vi "niRFUtil FTW Compute RBW and Sweep Time.vi"(0 "RBW Filter":T7={"Auto Bandwidth"=enum."True", "Type"=enum."Gaussian", "Bandwidth (Hz)"=100000.0, "Bandwidth Definition"=enum."3dB"} {"Bandwidth (Hz)" format="%^.3e"}, 5 "Sweep Time":T4={"Auto"=enum."True", "Interval (s)"=0.001} {"Interval (s)" format="%^.2e"}, 7 "FFT":T10={"Window"=enum."Flat Top", "Padding"=1.0} {"Padding" min=1.0 format="%.2f"}, 9 "IBW or Span (Hz)":dbl=1000000.0 format="%.3e", 12 "(IBW or Span)/RBW":dbl=100.0, 13 "RBW/Bin Size":dbl=10.0, 14 "Max DIBW (Hz)":dbl=inf format="%.3e") -> (3 "System RBW":T1={"Type"=enum."Gaussian", "Bandwidth (Hz)"=100000.0} {"Bandwidth (Hz)" format="%^.3e"}, 4 "RBW Filter Out":T7={"Auto Bandwidth"=enum."True", "Type"=enum."Gaussian", "Bandwidth (Hz)"=100000.0, "Bandwidth Definition"=enum."3dB"} {"Bandwidth (Hz)" format="%^.3e"}, 6 "Sweep Time Out":T4={"Auto"=enum."True", "Interval (s)"=0.001} {"Interval (s)" format="%^.2e"})   [LabVIEW 2015, in "niRFUtil.lvlib"]
uses:
  niRFUtil.lvlib
  Includes/niRFUtil INC RBW Filter (Freq Domain).ctl
  Includes/niRFUtil INC RBW Auto.ctl
  Includes/niRFUtil INC RBW Filter Type (Freq Domain).ctl
  Includes/niRFUtil INC RBW Filter Bandwidth.ctl
  Includes/niRFUtil INC Bandwidth Definition.ctl
  Includes/niRFUtil INC Sweep Time.ctl
  Includes/niRFUtil INC Sweep Time Auto.ctl
  Includes/niRFUtil INC Sweep Time Interval.ctl
  Includes/niRFUtil INC FFT.ctl
  Includes/niRFUtil INC FFT Window.ctl
  Includes/niRFUtil INC FFT Padding.ctl
  Includes/System/niRFUtil INC System RBW Filter (Frequency Domain).ctl
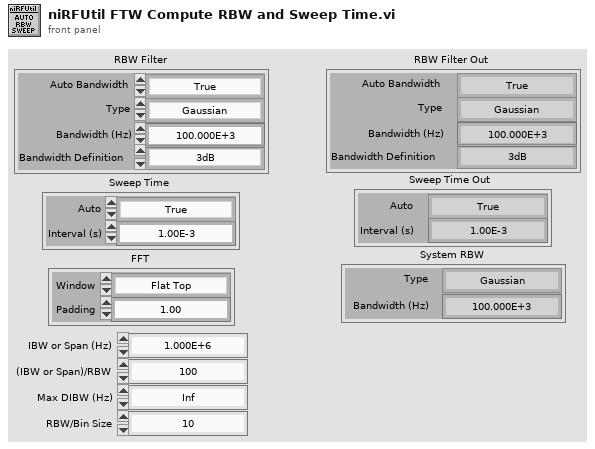
[diagram p1: front panel]
types:
  T1 = typedef "niRFUtil.lvlib/niRFUtil INC System RBW Filter (Frequency Domain).ctl" = cluster{"Type":T2, "Bandwidth (Hz)":T3}
  T2 = typedef "niRFUtil.lvlib/niRFUtil INC RBW Filter Type (Freq Domain).ctl" = enum16{"FFT Based", "Gaussian", "Flat", "Synch Tuned - 4", "Synch Tuned - 5"}
  T3 = typedef "niRFUtil.lvlib/niRFUtil INC RBW Filter Bandwidth.ctl" = dbl
  T4 = typedef "niRFUtil.lvlib/niRFUtil INC Sweep Time.ctl" = cluster{"Auto":T5, "Interval (s)":T6}
  T5 = typedef "niRFUtil.lvlib/niRFUtil INC Sweep Time Auto.ctl" = enum16{"False", "True"}
  T6 = typedef "niRFUtil.lvlib/niRFUtil INC Sweep Time Interval.ctl" = dbl
  T7 = typedef "niRFUtil.lvlib/niRFUtil INC RBW Filter (Freq Domain).ctl" = cluster{"Auto Bandwidth":T8, "Type":T2, "Bandwidth (Hz)":T3, "Bandwidth Definition":T9}
  T8 = typedef "niRFUtil.lvlib/niRFUtil INC RBW Auto.ctl" = enum16{"False", "True"}
  T9 = typedef "niRFUtil.lvlib/niRFUtil INC Bandwidth Definition.ctl" = enum16{"3dB", "6dB", "Bin Width", "ENBW"}
  T10 = typedef "niRFUtil.lvlib/niRFUtil INC FFT.ctl" = cluster{"Window":T11, "Padding":T12}
  T11 = typedef "niRFUtil.lvlib/niRFUtil INC FFT Window.ctl" = enum16{"None", "Flat Top", "Hanning", "Hamming", "Gaussian", "Blackman", "Blackman-Harris", "Kaiser-Bessel 70 dB", "Kaiser-Bessel 90 dB", "Kaiser-Bessel 110 dB"}
  T12 = typedef "niRFUtil.lvlib/niRFUtil INC FFT Padding.ctl" = dbl
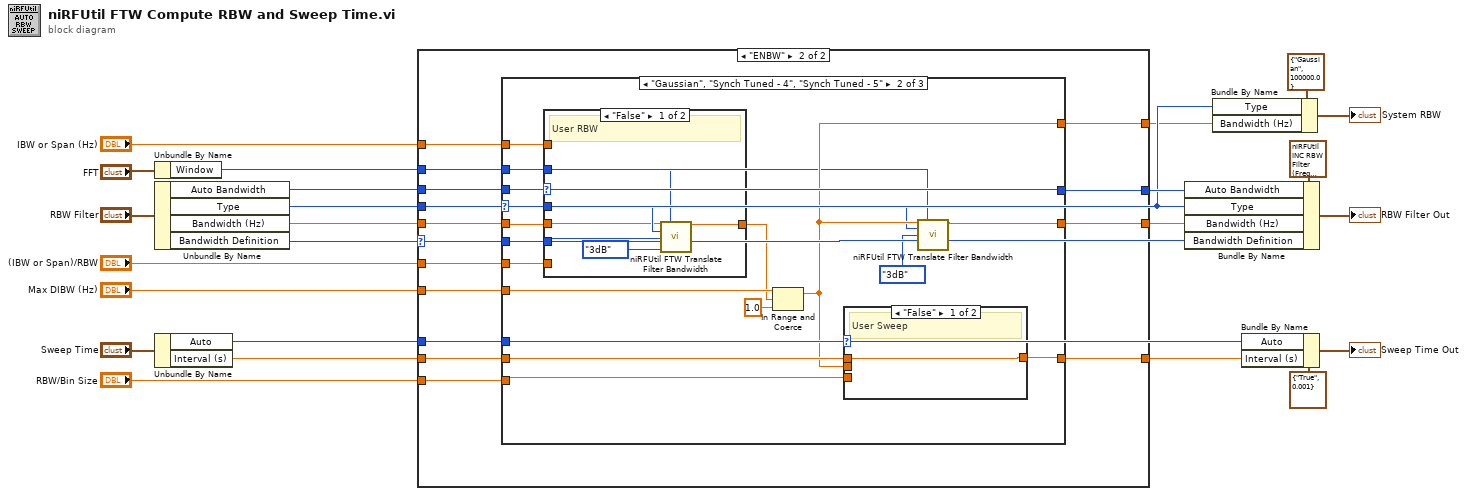
[diagram p0: block diagram]
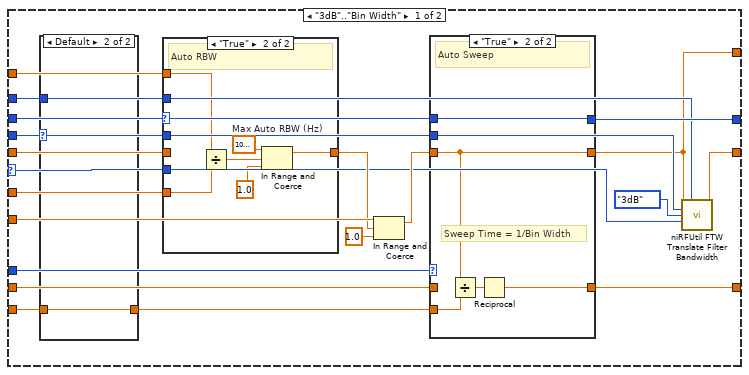
[diagram p2: hidden frame]
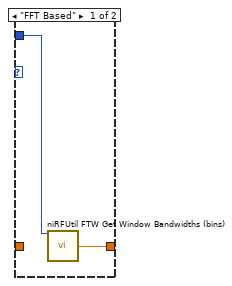
[diagram p3: hidden frame]
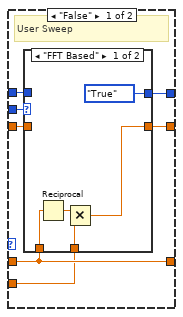
[diagram p4: hidden frame]
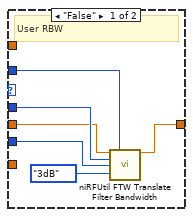
[diagram p6: hidden frame]
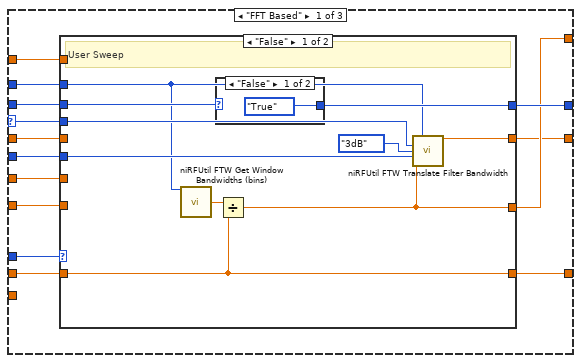
[diagram p7: hidden frame]
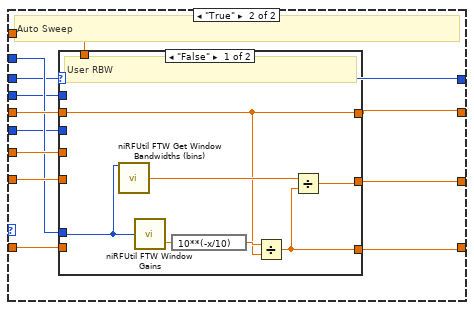
[diagram p9: hidden frame]
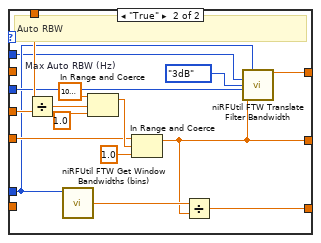
[diagram p10: hidden frame]
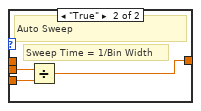
[diagram p11: hidden frame]
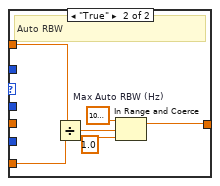
[diagram p12: hidden frame]
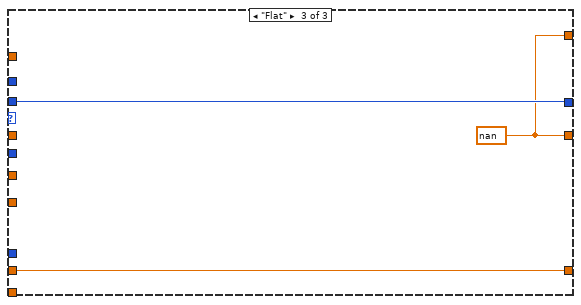
[diagram p13: hidden frame]
diagram:
  n1 = Unbundle By Name("FFT") -> ("Window"=w8:T11)
  n2 = Unbundle By Name("RBW Filter") -> ("Auto Bandwidth"=w10:T8, "Type"=w5:T2, "Bandwidth (Hz)"=w2:T3, "Bandwidth Definition"=w1:T9)
  n3 = Unbundle By Name("Sweep Time") -> ("Auto"=w3:T5, "Interval (s)"=w14:T6)
  n4 = case shown="\"ENBW\"" w1 {
    selector: w1 -> [w25 w79]
    tunnel: "IBW or Span (Hz)" -> [w44 w81]
    tunnel: "RBW/Bin Size" -> [w43 w82]
    tunnel: "(IBW or Span)/RBW" -> [w42 w84]
    tunnel: "Max DIBW (Hz)" -> [w41 w85]
    tunnel: w2 -> [w40 w80]
    tunnel: w14 -> [w39 w90]
    tunnel: w3 -> [w37 w91]
    tunnel: [w36 w89] -> w11
    tunnel: w10 -> [w35 w88]
    tunnel: [w34 w87] -> w9
    tunnel: w8 -> [w33 w92]
    tunnel: [w31 w83] -> w7
    tunnel: w5 -> [w30 w93]
    tunnel: [w29 w86] -> w4
    frame "3dB".."Bin Width" {
      n5 = case shown="Default" w30 {
        tunnel: w43 -> [_ w47]
        tunnel: [w46 w47] -> w38
        tunnel: w33 -> [w45 _]
        frame "FFT Based" {
          n6 = call "niRFUtil FTW Get Window Bandwidths (bins).vi"("FFT Window"=w45) -> ("Bins (3dB)"=w46:dbl)  [unwired: 12 in, 2 out]
        }
        frame Default {
        }
      }
      n7 = case shown="\"True\"" w35 {
        tunnel: [w68 w76] -> w28
        tunnel: w40 -> [w69 _]
        tunnel: w44 -> [_ w78]
        tunnel: w42 -> [_ w77]
        tunnel: w30 -> [w71 _]
        tunnel: w25 -> [w72 _]
        tunnel: w33 -> [w70 _]
        frame "False" {
          # "User RBW"
          n8 = call "niRFUtil FTW Translate Filter Bandwidth.vi"("Input Bandwidth (Hz)"=w69, "FFT Window"=w70, "Filter Type"=w71, "Input Bandwidth Definition"=w72, "Output Bandwidth Definition"=niRFUtil_INC_Bandwidth_Definition."3dB" ("Bandwidth Definition")) -> ("Output Bandwidth (Hz)"=w68:T3)  [unwired: 10 in]
        }
        frame "True" {
          w73 = 1000000.0  # Max Auto RBW (Hz)
          # "Auto RBW"
          n9 = Divide(x=w78, y=w77) -> (x/y=w75:dbl)
          n10 = In Range and Coerce(upper limit=w73, x=w75, lower limit=1.0) -> (coerced(x)=w76:dbl)  [unwired: 1 out]
        }
      }
      n11 = In Range and Coerce(upper limit=w41, x=w28, lower limit=1.0) -> (coerced(x)=w26:T3)  [unwired: 1 out]
      n12 = case shown="\"True\"" w37 {
        tunnel: w39 -> [w49 _]
        tunnel: w38 -> [w48 w66]
        tunnel: w26 -> [w51 w62]
        tunnel: [w49 w64] -> w36
        tunnel: w30 -> [w54 _]
        tunnel: w35 -> [w53 w63]
        tunnel: [w52 w63] -> w34
        tunnel: [w50 w62] -> w29
        frame "False" {
          # "User Sweep"
          n13 = case shown="\"FFT Based\"" w54 {
            tunnel: w53 -> [_ w61]
            tunnel: [niRFUtil_INC_RBW_Auto."True" ("Auto Bandwidth") w61] -> w52
            tunnel: w51 -> [_ w60]
            tunnel: [w55 w60] -> w50
            tunnel: w49 -> [w58 _]
            tunnel: w48 -> [w56 _]
            frame "FFT Based" {
              n14 = Reciprocal(x=w58) -> (1/x=w57:T6)
              n15 = Multiply(x=w57, y=w56) -> (x*y=w55:T6)
            }
            frame Default {
            }
          }
        }
        frame "True" {
          # "Sweep Time = 1/Bin Width"
          # "Auto Sweep"
          n16 = Divide(x=w62, y=w66) -> (x/y=w65:T3)
          n17 = Reciprocal(x=w65) -> (1/x=w64:T3)
        }
      }
      n18 = call "niRFUtil FTW Translate Filter Bandwidth.vi"("Input Bandwidth (Hz)"=w29, "FFT Window"=w33, "Filter Type"=w30, "Input Bandwidth Definition"=niRFUtil_INC_Bandwidth_Definition."3dB", "Output Bandwidth Definition"=w25) -> ("Output Bandwidth (Hz)"=w31:T3)  [unwired: 10 in]
    }
    frame "ENBW" {
      n19 = case shown="\"Gaussian\", \"Synch Tuned - 4\", \"Synch Tuned - 5\"" w93 {
        selector: w93 -> [w96 w155 _]
        tunnel: w92 -> [w102 w156 _]
        tunnel: w91 -> [w107 w167 _]
        tunnel: w90 -> [w106 w166 w188]
        tunnel: [w105 w165 w188] -> w89
        tunnel: w88 -> [w104 w161 w190]
        tunnel: [w103 w161 w190] -> w87
        tunnel: [w101 w158 w189] -> w86
        tunnel: w80 -> [w100 w168 _]
        tunnel: w85 -> [w99 w170 _]
        tunnel: w84 -> [w98 w162 _]
        tunnel: w79 -> [w97 w157 _]
        tunnel: [w95 w159 w189] -> w83
        tunnel: w82 -> [_ w164 _]
        tunnel: w81 -> [w94 w163 _]
        frame "FFT Based" {
          n20 = case shown="\"False\"" w107 {
            tunnel: [w115 w126] -> w105
            tunnel: w106 -> [w115 w125]
            tunnel: w104 -> [w117 w124]
            tunnel: w102 -> [w109 w128]
            tunnel: [w111 w124] -> w103
            tunnel: [w108 w127] -> w101
            tunnel: w100 -> [_ w131]
            tunnel: w99 -> [_ w129]
            tunnel: w98 -> [_ w130]
            tunnel: w97 -> [w113 w121]
            tunnel: w96 -> [w112 w120]
            tunnel: [w110 w122] -> w95
            tunnel: w94 -> [_ w123]
            frame "False" {
              # "User Sweep"
              n21 = call "niRFUtil FTW Get Window Bandwidths (bins).vi"("FFT Window"=w109) -> ("Bins (3dB)"=w116:dbl)  [unwired: 12 in, 2 out]
              n22 = case shown="\"False\"" w117 {
                selector: w117 -> [_ w119]
                tunnel: [niRFUtil_INC_RBW_Auto."True" ("Auto Bandwidth") w119] -> w111
                frame "False" {
                }
                frame "True" {
                  # "Auto RBW"
                }
              }
              n23 = Divide(x=w116, y=w115) -> (x/y=w108:T6)
              n24 = call "niRFUtil FTW Translate Filter Bandwidth.vi"("Input Bandwidth (Hz)"=w108, "FFT Window"=w109, "Filter Type"=w112, "Input Bandwidth Definition"=niRFUtil_INC_Bandwidth_Definition."3dB", "Output Bandwidth Definition"=w113) -> ("Output Bandwidth (Hz)"=w110:T3)  [unwired: 10 in]
            }
            frame "True" {
              # "Auto Sweep"
              n25 = case shown="\"False\"" w124 {
                tunnel: w131 -> [w133 _]
                tunnel: w130 -> [_ w151]
                tunnel: w129 -> [_ w148]
                tunnel: w128 -> [w135 w141]
                tunnel: [w134 w139] -> w127
                tunnel: [w132 w146] -> w126
                tunnel: w125 -> [_ _]
                tunnel: w123 -> [_ w145]
                tunnel: [w133 w143] -> w122
                tunnel: w121 -> [_ w142]
                tunnel: w120 -> [_ w140]
                frame "False" {
                  # "User RBW"
                  n26 = call "niRFUtil FTW Get Window Bandwidths (bins).vi"("FFT Window"=w135) -> ("Bins (3dB)"=w136:dbl)  [unwired: 12 in, 2 out]
                  n27 = call "niRFUtil FTW Window Gains.vi"("Window"=w135) -> ("-ENBW (dB-Hz)"=w138:sgl)  [unwired: 2 in, 1 out]
                  n28 = expression code="10**(-x/10)"(w138) -> (w137:sgl)
                  n29 = Divide(x=w137, y=w133) -> (x/y=w132:T3)
                  n30 = Divide(x=w136, y=w132) -> (x/y=w134:T3)
                }
                frame "True" {
                  w152 = 1000000.0  # Max Auto RBW (Hz)
                  # "Auto RBW"
                  n31 = Divide(x=w145, y=w151) -> (x/y=w154:dbl)
                  n32 = call "niRFUtil FTW Get Window Bandwidths (bins).vi"("FFT Window"=w141) -> ("Bins (3dB)"=w147:dbl)  [unwired: 12 in, 2 out]
                  n33 = In Range and Coerce(upper limit=w152, x=w154, lower limit=1.0) -> (coerced(x)=w149:dbl)  [unwired: 1 out]
                  n34 = In Range and Coerce(upper limit=w148, x=w149, lower limit=1.0) -> (coerced(x)=w139:dbl)  [unwired: 1 out]
                  n35 = Divide(x=w147, y=w139) -> (x/y=w146:dbl)
                  n36 = call "niRFUtil FTW Translate Filter Bandwidth.vi"("Input Bandwidth (Hz)"=w139, "FFT Window"=w141, "Filter Type"=w140, "Input Bandwidth Definition"=niRFUtil_INC_Bandwidth_Definition."3dB", "Output Bandwidth Definition"=w142) -> ("Output Bandwidth (Hz)"=w143:T3)  [unwired: 10 in]
                }
              }
            }
          }
        }
        frame "Gaussian", "Synch Tuned - 4", "Synch Tuned - 5" {
          n37 = case shown="\"False\"" w161 {
            tunnel: w168 -> [w177 _]
            tunnel: [w179 w182] -> w169
            tunnel: w157 -> [w180 _]
            tunnel: w155 -> [w178 _]
            tunnel: w156 -> [w176 _]
            tunnel: w163 -> [_ w184]
            tunnel: w162 -> [_ w183]
            frame "False" {
              # "User RBW"
              n38 = call "niRFUtil FTW Translate Filter Bandwidth.vi"("Input Bandwidth (Hz)"=w177, "FFT Window"=w176, "Filter Type"=w178, "Input Bandwidth Definition"=w180, "Output Bandwidth Definition"=niRFUtil_INC_Bandwidth_Definition."3dB" ("Input Bandwidth Definition")) -> ("Output Bandwidth (Hz)"=w179:T3)  [unwired: 10 in]
            }
            frame "True" {
              w185 = 1000000.0  # Max Auto RBW (Hz)
              # "Auto RBW"
              n39 = Divide(x=w184, y=w183) -> (x/y=w187:dbl)
              n40 = In Range and Coerce(upper limit=w185, x=w187, lower limit=1.0) -> (coerced(x)=w182:dbl)  [unwired: 1 out]
            }
          }
          n41 = In Range and Coerce(upper limit=w170, x=w169, lower limit=1.0) -> (coerced(x)=w158:T3)  [unwired: 1 out]
          n42 = case shown="\"False\"" w167 {
            tunnel: [w172 w173] -> w165
            tunnel: w166 -> [w172 _]
            tunnel: w164 -> [_ w175]
            tunnel: w158 -> [_ w174]
            frame "False" {
              # "User Sweep"
            }
            frame "True" {
              # "Sweep Time = 1/Bin Width"
              # "Auto Sweep"
              n43 = Divide(x=w175, y=w174) -> (x/y=w173:T3)
            }
          }
          n44 = call "niRFUtil FTW Translate Filter Bandwidth.vi"("Input Bandwidth (Hz)"=w158, "FFT Window"=w156, "Filter Type"=w155, "Input Bandwidth Definition"=niRFUtil_INC_Bandwidth_Definition."3dB", "Output Bandwidth Definition"=w157) -> ("Output Bandwidth (Hz)"=w159:T3)  [unwired: 10 in]
        }
        frame "Flat" {
          w189 = T3 nan ("Output Bandwidth (Hz)")
        }
      }
    }
  }
  n45 = Bundle By Name(cluster=T7 {"Auto Bandwidth"=enum."True", "Type"=enum."FFT Based", "Bandwidth (Hz)"=100000.0, "Bandwidth Definition"=enum."3dB"} ("RBW Filter Out"), "Auto Bandwidth"=w9, "Type"=w5, "Bandwidth (Hz)"=w7, "Bandwidth Definition"=w1) -> (→"RBW Filter Out":T7)
  n46 = Bundle By Name(cluster=T1 {"Type"=enum."Gaussian", "Bandwidth (Hz)"=100000.0} ("System RBW 2"), "Type"=w5, "Bandwidth (Hz)"=w4) -> (→"System RBW":T1)
  n47 = Bundle By Name(cluster=T4 {"Auto"=enum."True", "Interval (s)"=0.001} ("Sweep Time Out"), "Auto"=w3, "Interval (s)"=w11) -> (→"Sweep Time Out":T4)
